vi "Python String to LabVIEW Data (Variant).vi"(6 "Data Type (for skipping type check)":T1 format="%.0x", 8 "error in (no error)":errorcluster, 9 "type":variant, 10 "Python String":string) -> (0 "error out":errorcluster, 2 "LabVIEW Data":variant)   [LabVIEW 2020, in "jki_python_data_tools.lvlib"]
uses:
  jki_python_data_tools.lvlib
  <userlib>/_OpenG.lib/string/string.llb/openg_string.lvlib
  <userlib>/_OpenG.lib/lvdata/lvdata.llb/openg_variant.lvlib
  <userlib>/_OpenG.lib/error/error.llb/openg_error.lvlib
  <userlib>/_OpenG.lib/lvdata/lvdata.llb/Type Descriptor Enumeration__ogtk.ctl
panel:
  # "Copyright © 2003-2009 JKI. All rights reserved.\n\nAuthor:\nPhilippe Guerit [philippe.guerit@jameskring.com]\nJim Kring [jim.kring@jameskring.com]\n\nThis library is provided \"AS IS\" ,WITHOUT WARRANTIES OR \nCONDITIONS OF ANY KIND, either express or implied.\n\nJames Kring, Inc. -- http://www.jameskring.com"
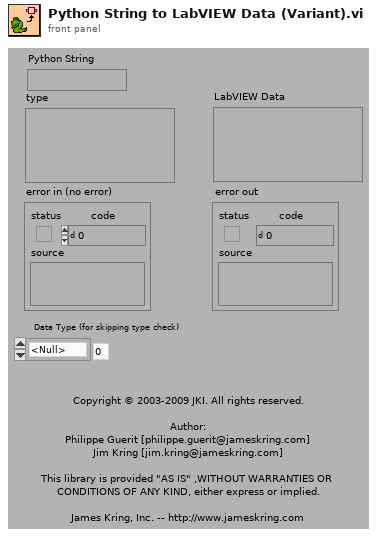
[diagram p1: front panel]
types:
  T1 = typedef "openg_variant.lvlib/Type Descriptor Enumeration__ogtk.ctl" = enum8{"<Null>", "I8", "I16", "I32", "I64", "U8", "U16", "U32", "U64", "SGL", "DBL", "EXT", "CSG", "CDB", "CXT", "0x0F", "0x10", "0x11", "0x12", "0x13", "0x14", "Enum U8", "Enum U16", "Enum U32", "Enum U64", "SGL PQ", "DBL PQ", "EXT PQ", "CSG PQ", "CDB PQ", "CXT PQ", "0x1F", "0x20", "Boolean", "0x22", "0x23", "0x24", "0x25", "0x26", "0x27", "0x28", "0x29", "0x2A", "0x2B", "0x2C", "0x2D", "0x2E", "0x2F", "String", "0x31", "Path", "Pict", "0x34", "0x35", "0x36", "DAQ", "0x38", "0x39", "0x3A", "0x3B", "0x3C", "0x3D", "0x3E", "0x3F", "Array", "0x41", "0x42", "0x43", "0x44", "0x45", "0x46", "0x47", "0x48", "0x49", "0x4A", "0x4B", "0x4C", "0x4D", "0x4E", "0x4F", "Cluster", "0x51", "0x52", "Variant", "Waveform", "0x55", "0x56", "0x57", "0x58", "0x59", "0x5A", "0x5B", "0x5C", "0x5D", "0x5E", "Fixed Point", "0x60", "0x61", "0x62", "0x63", "0x64", "0x65", "0x66", "0x67", "0x68", "0x69", "0x6A", "0x6B", "0x6C", "0x6D", "0x6E", "0x6F", "Refnum", "0x71", "0x72", "Set Collection", "Map Collection"}
  T2 = typedef "openg_variant.lvlib/Type Descriptor__ogtk.ctl" = i16[]
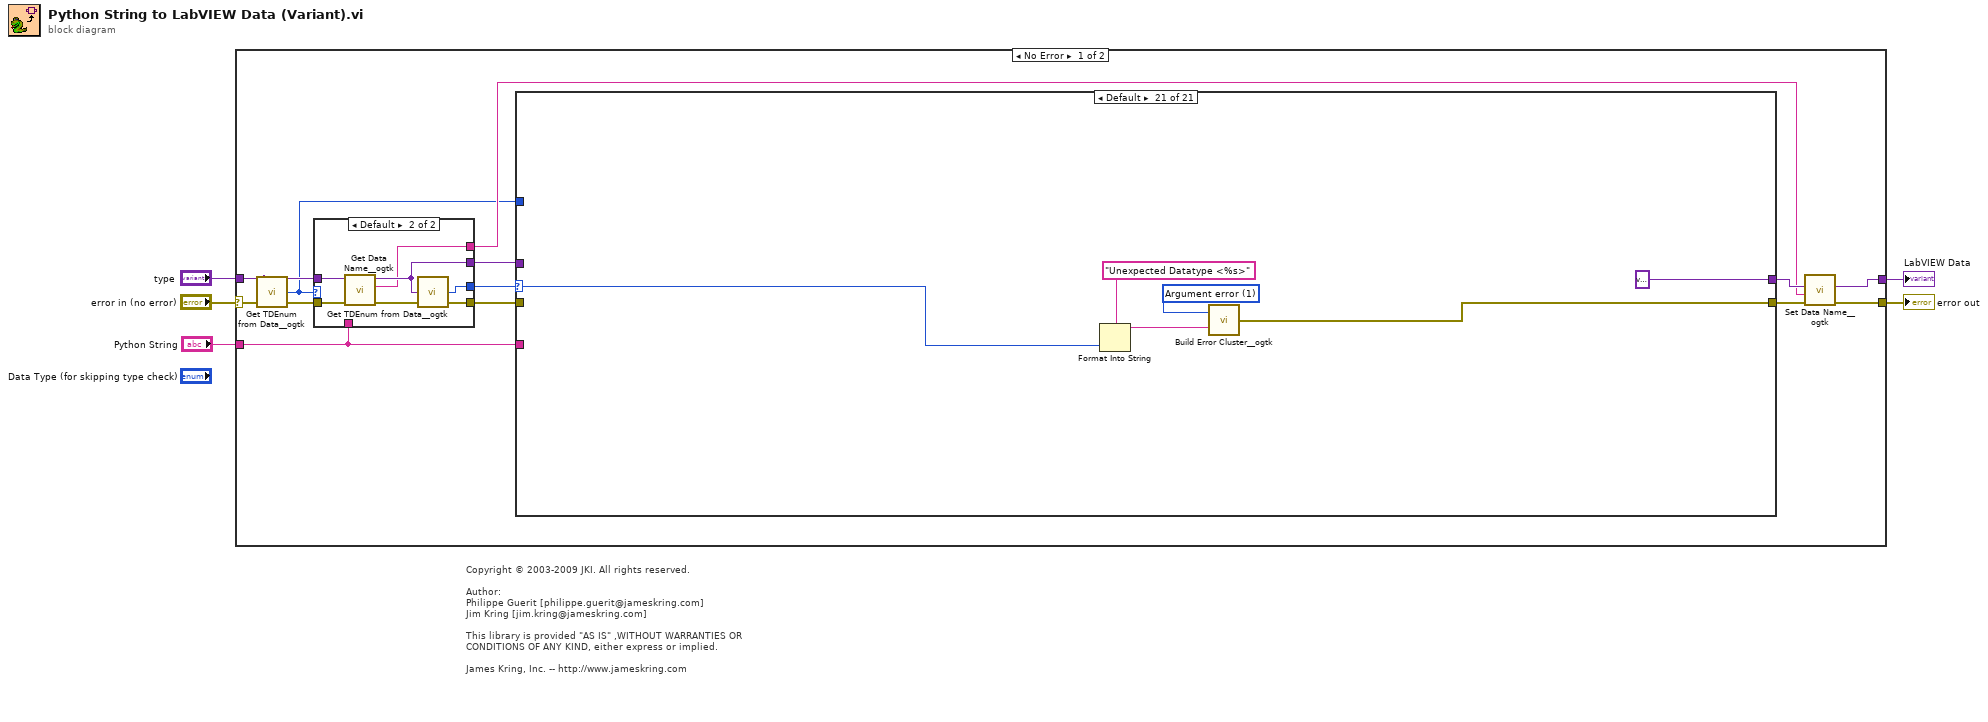
[diagram p0: block diagram]
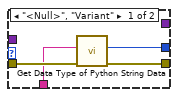
[diagram p2: hidden frame]
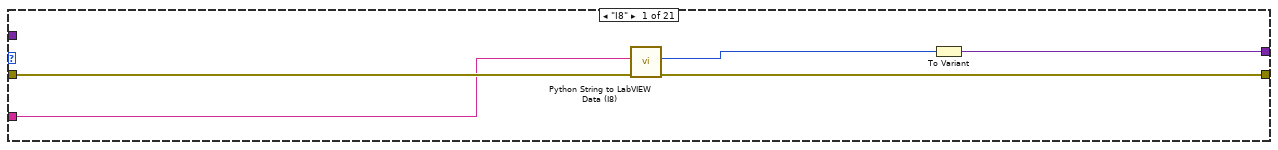
[diagram p3: hidden frame]
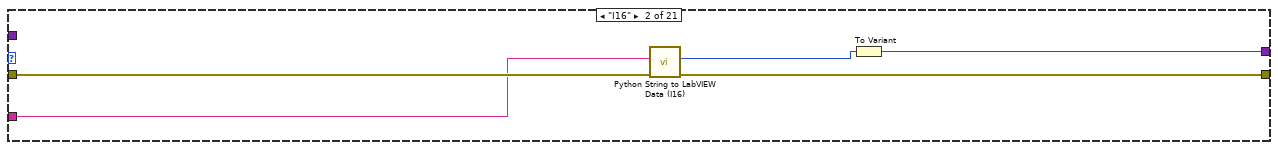
[diagram p4: hidden frame]
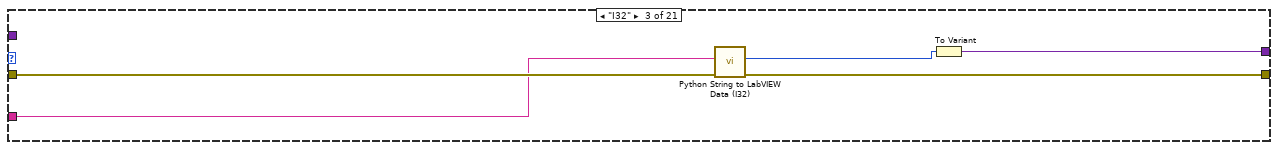
[diagram p5: hidden frame]
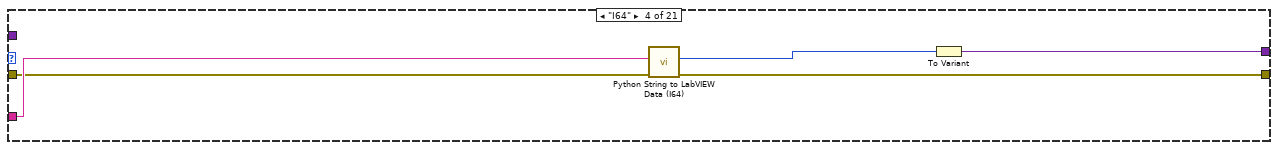
[diagram p6: hidden frame]
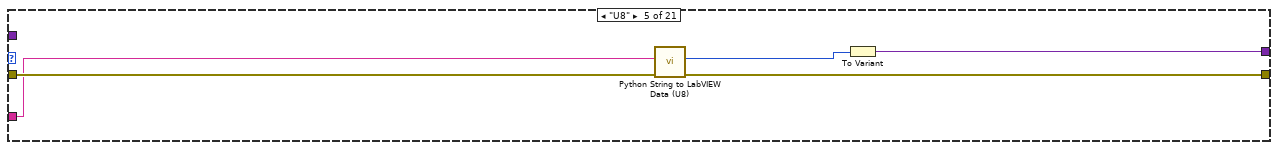
[diagram p7: hidden frame]
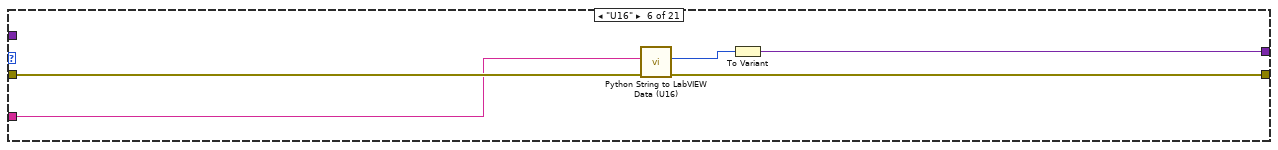
[diagram p8: hidden frame]
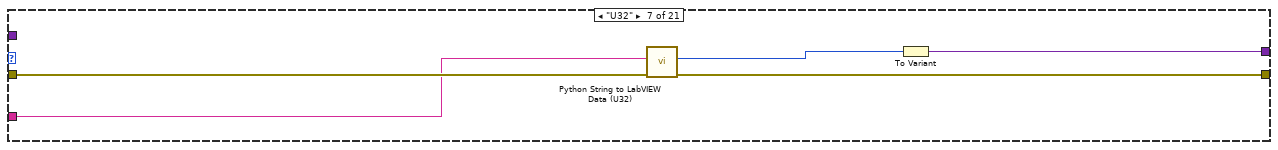
[diagram p9: hidden frame]
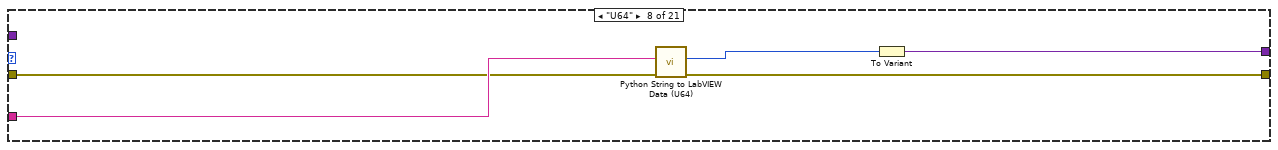
[diagram p10: hidden frame]
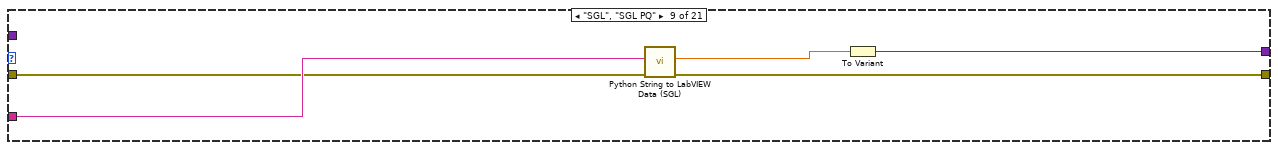
[diagram p11: hidden frame]
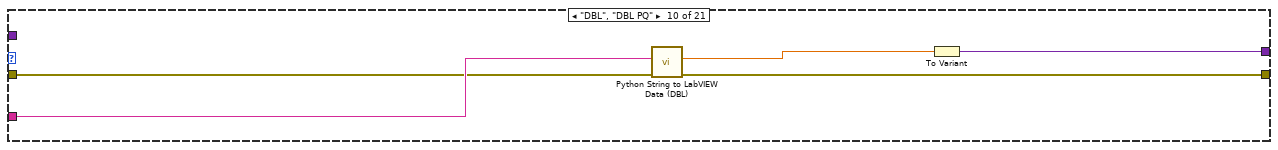
[diagram p12: hidden frame]
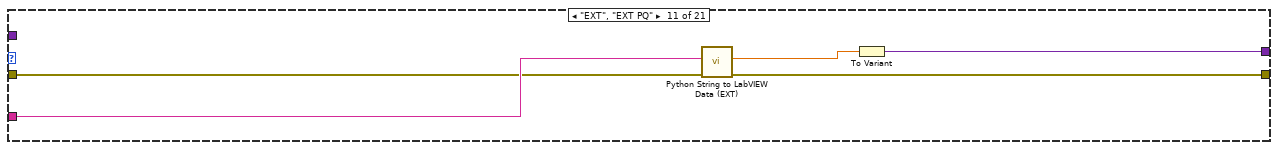
[diagram p13: hidden frame]
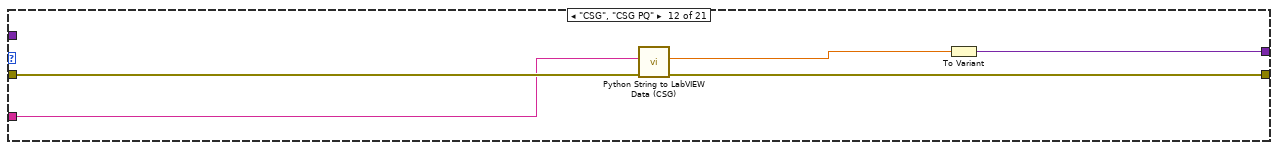
[diagram p14: hidden frame]
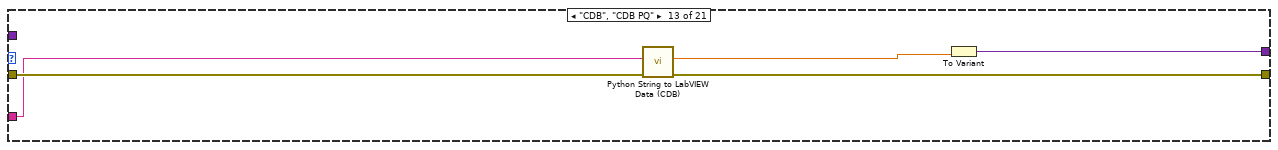
[diagram p15: hidden frame]
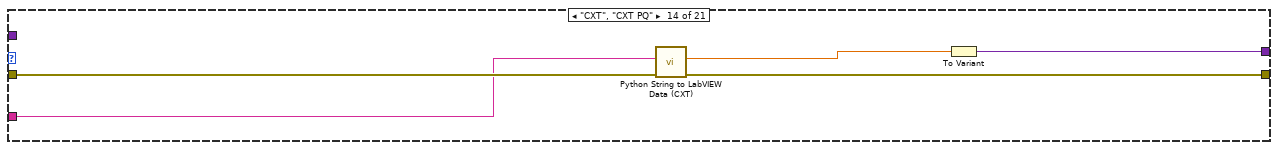
[diagram p16: hidden frame]
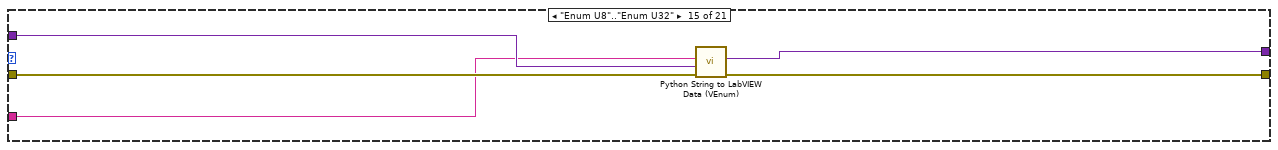
[diagram p17: hidden frame]
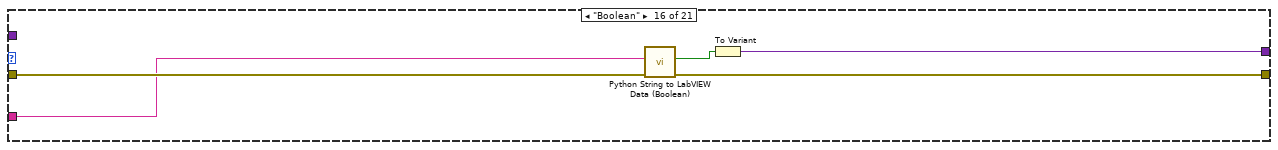
[diagram p18: hidden frame]
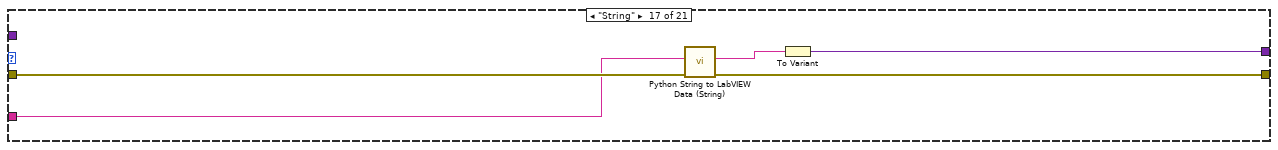
[diagram p19: hidden frame]
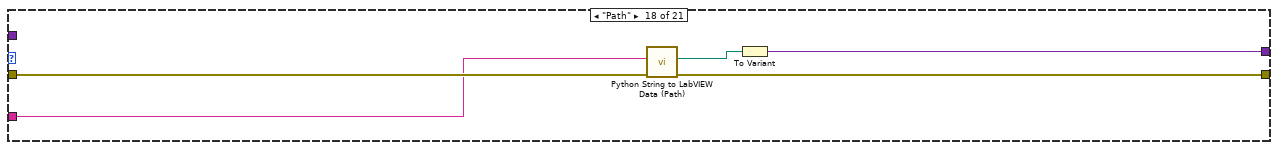
[diagram p20: hidden frame]
diagram:
  # "Copyright © 2003-2009 JKI. All rights reserved.\n\nAuthor:\nPhilippe Guerit [philippe.guerit@jameskring.com]\nJim Kring [jim.kring@jameskring.com]\n\nThis library is provided \"AS IS\" ,WITHOUT WARRANTIES OR \nCONDITIONS OF ANY KIND, either express or implied.\n\nJames Kring, Inc. -- http://www.jameskring.com"
  n1 = case shown="No Error" "error in (no error)" {
    selector: "error in (no error)" -> [w9 w756]
    tunnel: [w13 w756] -> w1
    tunnel: "type" -> [w8 _]
    tunnel: "Python String" -> [w7 _]
    tunnel: [w14 variant ("Variant")] -> w2
    frame No Error {
      n2 = call <userlib>:"Get TDEnum from Data__ogtk.vi"("Data"=w8) -> ("Type Descriptor Enumeration"=w6:T1)  [unwired: 4 in]
      n3 = case shown="Default" w6 {
        tunnel: [w18 w27] -> w17
        tunnel: [_ w26] -> w16
        tunnel: [w20 w25] -> w15
        tunnel: [_ w24] -> w10
        tunnel: w9 -> [w21 w23]
        tunnel: w8 -> [_ w22]
        tunnel: w7 -> [w19 _]
        frame "<Null>", "Variant" {
          n4 = call "Get Data Type of Python String Data.vi"("error in (no error)"=w21, "Python String"=w19) -> ("error out"=w20:errorcluster, "data type"=w18:T1)  [unwired: 8 in]
        }
        frame Default {
          n5 = call <userlib>:"Get Data Name__ogtk.vi"("error in (no error)"=w23, "Data"=w22) -> ("error out"=w25:errorcluster, "Data Name"=w24:string, "Data dup"=w26:variant)  [unwired: 7 in]
          n6 = call <userlib>:"Get TDEnum from Data__ogtk.vi"("Data"=w26) -> ("Type Descriptor Enumeration"=w27:T1)  [unwired: 4 in]
        }
      }
      n7 = case shown="Default" w17 {
        selector: w17 -> [_ _ _ _ _ _ _ _ _ _ _ _ _ _ _ _ _ _ _ _ w749]
        tunnel: w16 -> [_ _ _ _ _ _ _ _ _ _ _ _ _ _ w100 _ _ _ w121 w723 _]
        tunnel: [w30 w34 w40 w43 w48 w53 w60 w64 w70 w74 w79 w85 w89 w95 w101 w104 w108 w114 w119 w730 w753] -> w12
        tunnel: w15 -> [w32 w37 w41 w45 w51 w56 w61 w65 w68 w75 w80 w87 w92 w96 w102 w107 w112 w116 w120 w728 _]
        tunnel: [w31 w36 w42 w47 w52 w57 w62 w67 w72 w77 w82 w86 w91 w97 w99 w106 w111 w117 w118 w733 variant ("VCluster")] -> w11
        tunnel: w7 -> [w29 w33 w39 w46 w50 w55 w59 w66 w71 w76 w81 w83 w90 w94 w98 w105 w110 w113 w122 w729 _]
        tunnel: w6 -> [_ _ _ _ _ _ _ _ _ _ _ _ _ _ _ _ _ _ _ w725 _]
        frame "I8" {
          n8 = call "Python String to LabVIEW Data (I8).vi"("error in (no error)"=w32, "Python String"=w29) -> ("error out"=w30:errorcluster, "LabVIEW Data"=w28:i8)  [unwired: 8 in]
          n9 = To Variant(anything=w28) -> (Variant=w31:variant)
        }
        frame "I16" {
          n10 = call "Python String to LabVIEW Data (I16).vi"("error in (no error)"=w37, "Python String"=w33) -> ("error out"=w34:errorcluster, "LabVIEW Data"=w35:i16)  [unwired: 8 in]
          n11 = To Variant(anything=w35) -> (Variant=w36:variant)
        }
        frame "I32" {
          n12 = call "Python String to LabVIEW Data (I32).vi"("error in (no error)"=w41, "Python String"=w39) -> ("error out"=w40:errorcluster, "LabVIEW Data"=w38:i32)  [unwired: 8 in]
          n13 = To Variant(anything=w38) -> (Variant=w42:variant)
        }
        frame "I64" {
          n14 = call "Python String to LabVIEW Data (I64).vi"("error in (no error)"=w45, "Python String"=w46) -> ("error out"=w43:errorcluster, "LabVIEW Data"=w44:i64)  [unwired: 8 in]
          n15 = To Variant(anything=w44) -> (Variant=w47:variant)
        }
        frame "U8" {
          n16 = call "Python String to LabVIEW Data (U8).vi"("error in (no error)"=w51, "Python String"=w50) -> ("error out"=w48:errorcluster, "LabVIEW Data"=w49:u8)  [unwired: 8 in]
          n17 = To Variant(anything=w49) -> (Variant=w52:variant)
        }
        frame "U16" {
          n18 = call "Python String to LabVIEW Data (U16).vi"("error in (no error)"=w56, "Python String"=w55) -> ("error out"=w53:errorcluster, "LabVIEW Data"=w54:u16)  [unwired: 8 in]
          n19 = To Variant(anything=w54) -> (Variant=w57:variant)
        }
        frame "U32" {
          n20 = call "Python String to LabVIEW Data (U32).vi"("error in (no error)"=w61, "Python String"=w59) -> ("error out"=w60:errorcluster, "LabVIEW Data"=w58:u32)  [unwired: 8 in]
          n21 = To Variant(anything=w58) -> (Variant=w62:variant)
        }
        frame "U64" {
          n22 = call "Python String to LabVIEW Data (U64).vi"("error in (no error)"=w65, "Python String"=w66) -> ("error out"=w64:errorcluster, "LabVIEW Data"=w63:u64)  [unwired: 8 in]
          n23 = To Variant(anything=w63) -> (Variant=w67:variant)
        }
        frame "SGL", "SGL PQ" {
          n24 = call "Python String to LabVIEW Data (SGL).vi"("error in (no error)"=w68, "Python String"=w71) -> ("error out"=w70:errorcluster, "LabVIEW Data"=w69:sgl)  [unwired: 8 in]
          n25 = To Variant(anything=w69) -> (Variant=w72:variant)
        }
        frame "DBL", "DBL PQ" {
          n26 = call "Python String to LabVIEW Data (DBL).vi"("error in (no error)"=w75, "Python String"=w76) -> ("error out"=w74:errorcluster, "LabVIEW Data"=w73:dbl)  [unwired: 8 in]
          n27 = To Variant(anything=w73) -> (Variant=w77:variant)
        }
        frame "EXT", "EXT PQ" {
          n28 = call "Python String to LabVIEW Data (EXT).vi"("error in (no error)"=w80, "Python String"=w81) -> ("error out"=w79:errorcluster, "LabVIEW Data"=w78:ext)  [unwired: 8 in]
          n29 = To Variant(anything=w78) -> (Variant=w82:variant)
        }
        frame "CSG", "CSG PQ" {
          n30 = call "Python String to LabVIEW Data (CSG).vi"("error in (no error)"=w87, "Python String"=w83) -> ("error out"=w85:errorcluster, "LabVIEW Data"=w84:csg)  [unwired: 8 in]
          n31 = To Variant(anything=w84) -> (Variant=w86:variant)
        }
        frame "CDB", "CDB PQ" {
          n32 = call "Python String to LabVIEW Data (CDB).vi"("error in (no error)"=w92, "Python String"=w90) -> ("error out"=w89:errorcluster, "LabVIEW Data"=w88:cdb)  [unwired: 8 in]
          n33 = To Variant(anything=w88) -> (Variant=w91:variant)
        }
        frame "CXT", "CXT PQ" {
          n34 = call "Python String to LabVIEW Data (CXT).vi"("error in (no error)"=w96, "Python String"=w94) -> ("error out"=w95:errorcluster, "LabVIEW Data"=w93:cxt)  [unwired: 8 in]
          n35 = To Variant(anything=w93) -> (Variant=w97:variant)
        }
        frame "Enum U8".."Enum U32" {
          n36 = call "Python String to LabVIEW Data (VEnum).vi"("error in (no error)"=w102, "type (VEnum)"=w100, "Python String"=w98) -> ("error out"=w101:errorcluster, "LabVIEW Data"=w99:variant)  [unwired: 7 in]
        }
        frame "Boolean" {
          n37 = call "Python String to LabVIEW Data (Boolean).vi"("error in (no error)"=w107, "Python String"=w105) -> ("error out"=w104:errorcluster, "LabVIEW Data"=w103:bool)  [unwired: 8 in]
          n38 = To Variant(anything=w103) -> (Variant=w106:variant)
        }
        frame "String" {
          n39 = call "Python String to LabVIEW Data (String).vi"("error in (no error)"=w112, "Python String"=w110) -> ("error out"=w108:errorcluster, "LabVIEW Data"=w109:string)  [unwired: 8 in]
          n40 = To Variant(anything=w109) -> (Variant=w111:variant)
        }
        frame "Path" {
          n41 = call "Python String to LabVIEW Data (Path).vi"("error in (no error)"=w116, "Python String"=w113) -> ("error out"=w114:errorcluster, "LabVIEW Data"=w115:path)  [unwired: 8 in]
          n42 = To Variant(anything=w115) -> (Variant=w117:variant)
        }
        frame "Array" {
          n43 = disable-structure shown="Enabled" {
            disable-tunnel: w122 -> [w135 w166]
            disable-tunnel: w121 -> [w128 w170]
            disable-tunnel: w120 -> [w123 w174]
            disable-tunnel: [w125 w168] -> w119
            disable-tunnel: [w124 w167] -> w118
            frame Disabled {
              # "cluster or MutilD Array"
              # "Get Array Element\nvariant data type"
              # "/*Find opening \"[\" char*/"
              n44 = call <userlib>:"Get Array Element TDEnum__ogtk.vi"("error in (no error)"=w123, "Array"=w128) -> ("error out"=w134:errorcluster, "Element Type"=w126:T1)  [unwired: 8 in]
              n45 = call <userlib>:"Get Array Element TD__ogtk.vi"("error in (no error)"=w134, "Array"=w128) -> ("error out"=w133:errorcluster, "Type Descriptor"=w132:T2)  [unwired: 8 in]
              n46 = call "get text after first open bracket.vi"("Python String"=w135) -> ("Text After First Open Bracket"=w129:string)
              n47 = call <userlib>:"Get Default Data from TD__ogtk.vi"("error in (no error)"=w133, "Type Descriptor"=w132) -> ("error out"=w131:errorcluster, "Default VData"=w130:variant)  [unwired: 8 in]
              n48 = call "get text before last open bracket.vi"("Python String"=w129) -> ("Text After Last Open Bracket"=w127:string)
              n49 = case "Array Element Type" shown="\"Cluster\"" w126 {
                tunnel: w127 -> [w144 w160]
                tunnel: [w138 w157] -> w125
                tunnel: [w136 w156] -> w124
                tunnel: w130 -> [w137 w158]
                tunnel: w131 -> [w141 w159]
                frame "Cluster" {
                  n50 = call "Get Array Size from Python String.vi"("Python String"=w144) -> ("Array Size"=w142:i32, "Python String out"=w143:string)  [unwired: 9 in]
                  n51 = for "For each cluster element in the array" {
                    N: w142 -> [_]
                    tunnel: [w145] -> w140 mode=indexing
                    tunnel: w137 -> [w148]
                    shift-right: [w150] -> _
                    shift-left: w143 -> [w151]
                    shift-right: [w146] -> w139
                    shift-left: w141 -> [w147]
                    # "Recursive Call"
                    n52 = call "Split cluster or array pyhton string.vi"(11:w151) -> ("offset past element"=w150:i32, "First Element"=w149:string)  [unwired: 6 in, 3 out]
                    n53 = call "Python String to LabVIEW Data (Variant).vi"("error in (no error)"=w147, "type"=w148, "Python String"=w149) -> ("error out"=w146:errorcluster, "LabVIEW Data"=w145:variant)  [unwired: 7 in]
                  }
                  n54 = call <userlib>:"Array of VData to VArray__ogtk.vi"("error in (no error)"=w139, "Element Type (when empty)"=w137, "1D Array of VData"=w140) -> ("error out"=w138:errorcluster, "VArray"=w136:variant)  [unwired: 7 in]
                }
                frame Default {
                  # "Get Array Elements"
                  n55 = call <userlib>:"String to 1D Array__ogtk.vi"("delimiter (Tab)"=",", "string"=w160) -> ("Array of Strings"=w154:string[])  [unwired: 9 in]
                  n56 = for {
                    tunnel: w158 -> [w162]
                    tunnel: [w163] -> w153 mode=indexing
                    shift-right: [w164] -> w152
                    shift-left: w159 -> [w165]
                    tunnel: w154 -> [w161] mode=indexing
                    n57 = call "Python String to LabVIEW Data (Variant).vi"("error in (no error)"=w165, "type"=w162, "Python String"=w161) -> ("error out"=w164:errorcluster, "LabVIEW Data"=w163:variant)  [unwired: 7 in]
                  }
                  n58 = call <userlib>:"Array of VData to VArray__ogtk.vi"("error in (no error)"=w152, "Element Type (when empty)"=w158, "1D Array of VData"=w153) -> ("error out"=w157:errorcluster, "VArray"=w156:variant)  [unwired: 7 in]
                }
              }
            }
            frame Enabled {
              # "# of Dimensions"
              # "Get Array Element Type"
              n59 = call <userlib>:"Array Size(s)__ogtk.vi"("error in (no error)"=w174, "Array"=w170) -> ("error out"=w172:errorcluster, "N dims"=w173:u32)  [unwired: 7 in, 1 out]
              n60 = call <userlib>:"Get Array Element TDEnum__ogtk.vi"("error in (no error)"=w172, "Array"=w170) -> ("error out"=w171:errorcluster, "Element Type"=w169:T1)  [unwired: 8 in]
              n61 = case "Array dimension" shown="Default" w173 {
                tunnel: w170 -> [w181 w219 w368]
                tunnel: w171 -> [w176 w216 w363]
                tunnel: w169 -> [w182 w220 w369]
                tunnel: w166 -> [w178 w215 w365]
                tunnel: [w180 w218 w367] -> w168
                tunnel: [w179 w217 w366] -> w167
                frame Default {
                  # "Array of dim >= 2\nare not supported so put default code (that will failed) here for all array dim greater to 2"
                  n62 = call "Python List to Array of Elements.vi"("error in (no error)"=w176, "Python List"=w178) -> ("error out"=w175:errorcluster, "Elements"=w177:string[])  [unwired: 8 in]
                  n63 = case shown="Default" w182 {
                    tunnel: w175 -> [w187 w206]
                    tunnel: w181 -> [w185 w205]
                    tunnel: w177 -> [w183 w209]
                    tunnel: [w191 w199] -> w180
                    tunnel: [w190 w200] -> w179
                    frame Default {
                      # "Get Array Element\nvariant data type"
                      n64 = call <userlib>:"Get Array Element TD__ogtk.vi"("error in (no error)"=w187, "Array"=w185) -> ("error out"=w189:errorcluster, "Type Descriptor"=w188:T2)  [unwired: 8 in]
                      n65 = call <userlib>:"Get Default Data from TD__ogtk.vi"("error in (no error)"=w189, "Type Descriptor"=w188) -> ("error out"=w186:errorcluster, "Default VData"=w184:variant)  [unwired: 8 in]
                      n66 = for {
                        tunnel: w184 -> [w195]
                        tunnel: [w196] -> w193 mode=indexing
                        shift-right: [w197] -> w192
                        shift-left: w186 -> [w198]
                        tunnel: w183 -> [w194] mode=indexing
                        n67 = call "Python String to LabVIEW Data (Variant).vi"("error in (no error)"=w198, "type"=w195, "Python String"=w194) -> ("error out"=w197:errorcluster, "LabVIEW Data"=w196:variant)  [unwired: 7 in]
                      }
                      n68 = call <userlib>:"Array of VData to VArray__ogtk.vi"("error in (no error)"=w192, "Element Type (when empty)"=w184, "1D Array of VData"=w193) -> ("error out"=w191:errorcluster, "VArray"=w190:variant)  [unwired: 7 in]
                    }
                    frame "Cluster" {
                      # "Get Array Element\nvariant data type"
                      n69 = call <userlib>:"Get Array Element TD__ogtk.vi"("error in (no error)"=w206, "Array"=w205) -> ("error out"=w208:errorcluster, "Type Descriptor"=w207:T2)  [unwired: 8 in]
                      n70 = call <userlib>:"Get Default Data from TD__ogtk.vi"("error in (no error)"=w208, "Type Descriptor"=w207) -> ("error out"=w204:errorcluster, "Default VData"=w201:variant)  [unwired: 8 in]
                      n71 = for "For each cluster element in the array" {
                        tunnel: [w212] -> w202 mode=indexing
                        tunnel: w201 -> [w214]
                        shift-right: [w213] -> w203
                        shift-left: w204 -> [w210]
                        tunnel: w209 -> [w211] mode=indexing
                        # "Recursive Call"
                        n72 = call "Python String to LabVIEW Data (Variant).vi"("error in (no error)"=w210, "type"=w214, "Python String"=w211) -> ("error out"=w213:errorcluster, "LabVIEW Data"=w212:variant)  [unwired: 7 in]
                      }
                      n73 = call <userlib>:"Array of VData to VArray__ogtk.vi"("error in (no error)"=w203, "Element Type (when empty)"=w201, "1D Array of VData"=w202) -> ("error out"=w199:errorcluster, "VArray"=w200:variant)  [unwired: 7 in]
                    }
                  }
                }
                frame 1 {
                  # "1D array"
                  n74 = case shown="\"Cluster\"" w220 {
                    tunnel: w216 -> [w227 w243 w248 w251 w257 w262 w268 w272 w277 w282 w287 w292 w297 w302 w307 w313 w318 w323 w334]
                    tunnel: w219 -> [w226 _ _ _ _ _ _ _ _ _ _ _ _ _ _ _ _ _ w333]
                    tunnel: w215 -> [w224 w239 w244 w250 w256 w261 w264 w269 w274 w279 w284 w289 w294 w299 w304 w309 w314 w319 w327]
                    tunnel: [w231 w242 w247 w252 w258 w263 w267 w271 w276 w281 w286 w291 w296 w301 w306 w312 w317 w322 w328] -> w218
                    tunnel: [w230 w240 w245 w253 w254 w259 w265 w273 w278 w283 w288 w293 w298 w303 w308 w310 w315 w320 w329] -> w217
                    frame Default {
                      # "Get Array Element\nvariant data type"
                      n75 = call <userlib>:"Get Array Element TD__ogtk.vi"("error in (no error)"=w227, "Array"=w226) -> ("error out"=w229:errorcluster, "Type Descriptor"=w228:T2)  [unwired: 8 in]
                      n76 = call <userlib>:"Get Default Data from TD__ogtk.vi"("error in (no error)"=w229, "Type Descriptor"=w228) -> ("error out"=w222:errorcluster, "Default VData"=w225:variant)  [unwired: 8 in]
                      n77 = call "Python List to Array of Elements.vi"("error in (no error)"=w222, "Python List"=w224) -> ("error out"=w221:errorcluster, "Elements"=w223:string[])  [unwired: 8 in]
                      n78 = for {
                        tunnel: w225 -> [w235]
                        tunnel: [w236] -> w233 mode=indexing
                        shift-right: [w237] -> w232
                        shift-left: w221 -> [w238]
                        tunnel: w223 -> [w234] mode=indexing
                        n79 = call "Python String to LabVIEW Data (Variant).vi"("error in (no error)"=w238, "type"=w235, "Python String"=w234) -> ("error out"=w237:errorcluster, "LabVIEW Data"=w236:variant)  [unwired: 7 in]
                      }
                      n80 = call <userlib>:"Array of VData to VArray__ogtk.vi"("error in (no error)"=w232, "Element Type (when empty)"=w225, "1D Array of VData"=w233) -> ("error out"=w231:errorcluster, "VArray"=w230:variant)  [unwired: 7 in]
                    }
                    frame "I8" {
                      n81 = call "Python String to LabVIEW Data (I8 Array).vi"("error in (no error)"=w243, "Python String"=w239) -> ("error out"=w242:errorcluster, "LabVIEW Data"=w241:i8[])  [unwired: 8 in]
                      n82 = To Variant(anything=w241) -> (Variant=w240:variant)
                    }
                    frame "I16" {
                      n83 = call "Python String to LabVIEW Data (I16 Array).vi"("error in (no error)"=w248, "Python String"=w244) -> ("error out"=w247:errorcluster, "LabVIEW Data"=w246:i16[])  [unwired: 8 in]
                      n84 = To Variant(anything=w246) -> (Variant=w245:variant)
                    }
                    frame "I32" {
                      n85 = call "Python String to LabVIEW Data (I32 Array).vi"("error in (no error)"=w251, "Python String"=w250) -> ("error out"=w252:errorcluster, "LabVIEW Data"=w249:i32[])  [unwired: 8 in]
                      n86 = To Variant(anything=w249) -> (Variant=w253:variant)
                    }
                    frame "I64" {
                      n87 = call "Python String to LabVIEW Data (I64 Array).vi"("error in (no error)"=w257, "Python String"=w256) -> ("error out"=w258:errorcluster, "LabVIEW Data"=w255:i64[])  [unwired: 8 in]
                      n88 = To Variant(anything=w255) -> (Variant=w254:variant)
                    }
                    frame "U8" {
                      n89 = call "Python String to LabVIEW Data (U8 Array).vi"("error in (no error)"=w262, "Python String"=w261) -> ("error out"=w263:errorcluster, "LabVIEW Data"=w260:u8[])  [unwired: 8 in]
                      n90 = To Variant(anything=w260) -> (Variant=w259:variant)
                    }
                    frame "U16" {
                      n91 = call "Python String to LabVIEW Data (U16 Array).vi"("error in (no error)"=w268, "Python String"=w264) -> ("error out"=w267:errorcluster, "LabVIEW Data"=w266:u16[])  [unwired: 8 in]
                      n92 = To Variant(anything=w266) -> (Variant=w265:variant)
                    }
                    frame "U32" {
                      n93 = call "Python String to LabVIEW Data (U32 Array).vi"("error in (no error)"=w272, "Python String"=w269) -> ("error out"=w271:errorcluster, "LabVIEW Data"=w270:u32[])  [unwired: 8 in]
                      n94 = To Variant(anything=w270) -> (Variant=w273:variant)
                    }
                    frame "U64" {
                      n95 = call "Python String to LabVIEW Data (U64 Array).vi"("error in (no error)"=w277, "Python String"=w274) -> ("error out"=w276:errorcluster, "LabVIEW Data"=w275:u64[])  [unwired: 8 in]
                      n96 = To Variant(anything=w275) -> (Variant=w278:variant)
                    }
                    frame "SGL", "SGL PQ" {
                      n97 = call "Python String to LabVIEW Data (SGL Array).vi"("error in (no error)"=w282, "Python String"=w279) -> ("error out"=w281:errorcluster, "LabVIEW Data"=w280:sgl[])  [unwired: 8 in]
                      n98 = To Variant(anything=w280) -> (Variant=w283:variant)
                    }
                    frame "DBL", "DBL PQ" {
                      n99 = call "Python String to LabVIEW Data (DBL Array).vi"("error in (no error)"=w287, "Python String"=w284) -> ("error out"=w286:errorcluster, "LabVIEW Data"=w285:dbl[])  [unwired: 8 in]
                      n100 = To Variant(anything=w285) -> (Variant=w288:variant)
                    }
                    frame "EXT", "EXT PQ" {
                      n101 = call "Python String to LabVIEW Data (EXT Array).vi"("error in (no error)"=w292, "Python String"=w289) -> ("error out"=w291:errorcluster, "LabVIEW Data"=w290:ext[])  [unwired: 8 in]
                      n102 = To Variant(anything=w290) -> (Variant=w293:variant)
                    }
                    frame "CSG", "CSG PQ" {
                      n103 = call "Python String to LabVIEW Data (CSG Array).vi"("error in (no error)"=w297, "Python String"=w294) -> ("error out"=w296:errorcluster, "LabVIEW Data"=w295:csg[])  [unwired: 8 in]
                      n104 = To Variant(anything=w295) -> (Variant=w298:variant)
                    }
                    frame "CDB", "CDB PQ" {
                      n105 = call "Python String to LabVIEW Data (CDB Array).vi"("error in (no error)"=w302, "Python String"=w299) -> ("error out"=w301:errorcluster, "LabVIEW Data"=w300:cdb[])  [unwired: 8 in]
                      n106 = To Variant(anything=w300) -> (Variant=w303:variant)
                    }
                    frame "CXT", "CXT PQ" {
                      n107 = call "Python String to LabVIEW Data (CXT Array).vi"("error in (no error)"=w307, "Python String"=w304) -> ("error out"=w306:errorcluster, "LabVIEW Data"=w305:cxt[])  [unwired: 8 in]
                      n108 = To Variant(anything=w305) -> (Variant=w308:variant)
                    }
                    frame "Boolean" {
                      n109 = call "Python String to LabVIEW Data (Boolean Array).vi"("error in (no error)"=w313, "Python String"=w309) -> ("error out"=w312:errorcluster, "LabVIEW Data"=w311:bool[])  [unwired: 8 in]
                      n110 = To Variant(anything=w311) -> (Variant=w310:variant)
                    }
                    frame "String" {
                      n111 = call "Python String to LabVIEW Data (String Array).vi"("error in (no error)"=w318, "Python String"=w314) -> ("error out"=w317:errorcluster, "LabVIEW Data"=w316:string[])  [unwired: 8 in]
                      n112 = To Variant(anything=w316) -> (Variant=w315:variant)
                    }
                    frame "Path" {
                      n113 = call "Python String to LabVIEW Data (Path Array).vi"("error in (no error)"=w323, "Python String"=w319) -> ("error out"=w322:errorcluster, "LabVIEW Data"=w321:path[])  [unwired: 8 in]
                      n114 = To Variant(anything=w321) -> (Variant=w320:variant)
                    }
                    frame "Cluster" {
                      # "Get Array Element\nvariant data type"
                      n115 = call <userlib>:"Get Array Element TD__ogtk.vi"("error in (no error)"=w334, "Array"=w333) -> ("error out"=w336:errorcluster, "Type Descriptor"=w335:T2)  [unwired: 8 in]
                      n116 = call <userlib>:"Get Default Data from TD__ogtk.vi"("error in (no error)"=w336, "Type Descriptor"=w335) -> ("error out"=w325:errorcluster, "Default VData"=w330:variant)  [unwired: 8 in]
                      n117 = call "Python List to Array of Elements.vi"("error in (no error)"=w325, "Python List"=w327) -> ("error out"=w324:errorcluster, "Elements"=w326:string[])  [unwired: 8 in]
                      n118 = disable-structure shown="Disabled" {
                        disable-tunnel: w326 -> [w342 w352 _]
                        disable-tunnel: w324 -> [w341 w356 _]
                        disable-tunnel: [w340 w355 _] -> w332
                        disable-tunnel: [w339 w354 _] -> w331
                        disable-tunnel: w330 -> [w338 w353 _]
                        frame Disabled {
                          n119 = call "get text between brackets.vi"("Python String"=w342) -> ("Text Between Brakets"=w337:string)  [unwired: 10 in]
                          n120 = call "Get Array Size from Python String.vi"("Python String"=w337) -> ("Array Size"=w343:i32, "Python String out"=w344:string)  [unwired: 9 in]
                          n121 = for "For each cluster element in the array" {
                            N: w343 -> [_]
                            tunnel: [w345] -> w339 mode=indexing
                            tunnel: w338 -> [w348]
                            shift-right: [w350] -> _
                            shift-left: w344 -> [w351]
                            shift-right: [w346] -> w340
                            shift-left: w341 -> [w347]
                            # "Recursive Call"
                            n122 = call "Split cluster or array pyhton string.vi"(11:w351) -> ("offset past element"=w350:i32, "First Element"=w349:string)  [unwired: 6 in, 3 out]
                            n123 = call "Python String to LabVIEW Data (Variant).vi"("error in (no error)"=w347, "type"=w348, "Python String"=w349) -> ("error out"=w346:errorcluster, "LabVIEW Data"=w345:variant)  [unwired: 7 in]
                          }
                        }
                        frame Enabled {
                          n124 = for "For each cluster element in the array" {
                            tunnel: [w359] -> w354 mode=indexing
                            tunnel: w353 -> [w361]
                            shift-right: [w360] -> w355
                            shift-left: w356 -> [w357]
                            tunnel: w352 -> [w358] mode=indexing
                            # "Recursive Call"
                            n125 = call "Python String to LabVIEW Data (Variant).vi"("error in (no error)"=w357, "type"=w361, "Python String"=w358) -> ("error out"=w360:errorcluster, "LabVIEW Data"=w359:variant)  [unwired: 7 in]
                          }
                        }
                        frame Disabled {
                        }
                      }
                      n126 = call <userlib>:"Array of VData to VArray__ogtk.vi"("error in (no error)"=w332, "Element Type (when empty)"=w330, "1D Array of VData"=w331) -> ("error out"=w328:errorcluster, "VArray"=w329:variant)  [unwired: 7 in]
                    }
                  }
                }
                frame 2 {
                  # "2D array"
                  n127 = call "Python List to Array of Elements.vi"("error in (no error)"=w363, "Python List"=w365) -> ("error out"=w362:errorcluster, "Elements"=w364:string[])  [unwired: 8 in]
                  n128 = case shown="\"I8\"" w369 {
                    tunnel: w362 -> [w380 w395 w409 w429 w446 w463 w480 w497 w514 w531 w548 w565 w582 w599 w616 w633 w650 w667 w688]
                    tunnel: w368 -> [w379 _ _ _ _ _ _ _ _ _ _ _ _ _ _ _ _ _ w687]
                    tunnel: [w377 w394 w412 w428 w445 w462 w479 w496 w513 w530 w547 w564 w581 w598 w615 w632 w649 w666 w684] -> w367
                    tunnel: [w376 w392 w410 w426 w443 w460 w477 w494 w511 w528 w545 w562 w579 w596 w613 w630 w647 w664 w682] -> w366
                    tunnel: w364 -> [w370 w391 w408 w425 w442 w459 w476 w493 w510 w527 w544 w561 w578 w595 w612 w629 w646 w663 w681]
                    frame Default {
                      # "Get Array Element\nvariant data type"
                      n129 = call <userlib>:"Get Array Element TD__ogtk.vi"("error in (no error)"=w380, "Array"=w379) -> ("error out"=w382:errorcluster, "Type Descriptor"=w381:T2)  [unwired: 8 in]
                      n130 = call <userlib>:"Get Default Data from TD__ogtk.vi"("error in (no error)"=w382, "Type Descriptor"=w381) -> ("error out"=w371:errorcluster, "Default VData"=w374:variant)  [unwired: 8 in]
                      n131 = Build Array(w374) -> (w375:variant[])
                      n132 = call <userlib>:"Array of VData to VArray__ogtk.vi"("error in (no error)"=w371, "Element Type (when empty)"=w374, "1D Array of VData"=w375) -> ("error out"=w372:errorcluster, "VArray"=w373:variant)  [unwired: 7 in]
                      n133 = for {
                        tunnel: w373 -> [w389]
                        shift-right: [w386] -> w377
                        shift-left: w372 -> [w390]
                        tunnel: [w384] -> w378 mode=indexing
                        tunnel: w370 -> [w383] mode=indexing
                        n134 = call "Python String to LabVIEW Data (Variant).vi"("error in (no error)"=w390, "type"=w389, "Python String"=w383) -> ("error out"=w387:errorcluster, "LabVIEW Data"=w388:variant)  [unwired: 7 in]
                        n135 = Variant To Data(error in=w387, type=variant[] [], Variant=w388) -> (data=w384:variant[], error out=w386:errorcluster)
                      }
                      n136 = To Variant(anything=w378) -> (Variant=w376:variant)
                    }
                    frame "I8" {
                      n137 = for {
                        tunnel: [w401] -> w393 mode=indexing
                        shift-right: [w402] -> w394
                        shift-left: w395 -> [w398]
                        tunnel: w391 -> [w397] mode=indexing
                        # "Get Array Elements"
                        n138 = call "get text between brackets.vi"("Python String"=w397) -> ("Text Between Brakets"=w396:string)  [unwired: 10 in]
                        n139 = call <userlib>:"String to 1D Array__ogtk.vi"("delimiter (Tab)"=",", "string"=w396) -> ("Array of Strings"=w399:string[])  [unwired: 9 in]
                        n140 = for {
                          tunnel: [w403] -> w401 mode=indexing
                          tunnel: w399 -> [w404] mode=indexing
                          shift-right: [w406] -> w402
                          shift-left: w398 -> [w407]
                          w405 = i8 0  # I8 Type
                          n141 = Scan From String(input string=w404, error in=w407, default 1=w405) -> (error out=w406:errorcluster, output 1=w403:i8)  [unwired: 2 in, 2 out]
                        }
                      }
                      n142 = To Variant(anything=w393) -> (Variant=w392:variant)
                    }
                    frame "I16" {
                      n143 = for {
                        tunnel: [w417] -> w411 mode=indexing
                        tunnel: w408 -> [w414] mode=indexing
                        shift-right: [w418] -> w412
                        shift-left: w409 -> [w419]
                        # "Get Array Elements"
                        n144 = call "get text between brackets.vi"("Python String"=w414) -> ("Text Between Brakets"=w413:string)  [unwired: 10 in]
                        n145 = call <userlib>:"String to 1D Array__ogtk.vi"("delimiter (Tab)"=",", "string"=w413) -> ("Array of Strings"=w415:string[])  [unwired: 9 in]
                        n146 = for {
                          tunnel: [w420] -> w417 mode=indexing
                          tunnel: w415 -> [w421] mode=indexing
                          shift-right: [w423] -> w418
                          shift-left: w419 -> [w424]
                          w422 = i16 0  # I16 Type
                          n147 = Scan From String(input string=w421, error in=w424, default 1=w422) -> (error out=w423:errorcluster, output 1=w420:i16)  [unwired: 2 in, 2 out]
                        }
                      }
                      n148 = To Variant(anything=w411) -> (Variant=w410:variant)
                    }
                    frame "I32" {
                      n149 = for {
                        tunnel: [w434] -> w427 mode=indexing
                        tunnel: w425 -> [w431] mode=indexing
                        shift-right: [w435] -> w428
                        shift-left: w429 -> [w436]
                        # "Get Array Elements"
                        n150 = call "get text between brackets.vi"("Python String"=w431) -> ("Text Between Brakets"=w430:string)  [unwired: 10 in]
                        n151 = call <userlib>:"String to 1D Array__ogtk.vi"("delimiter (Tab)"=",", "string"=w430) -> ("Array of Strings"=w432:string[])  [unwired: 9 in]
                        n152 = for {
                          tunnel: [w437] -> w434 mode=indexing
                          tunnel: w432 -> [w438] mode=indexing
                          shift-right: [w440] -> w435
                          shift-left: w436 -> [w441]
                          w439 = 0  # I32 Type
                          n153 = Scan From String(input string=w438, error in=w441, default 1=w439) -> (error out=w440:errorcluster, output 1=w437:i32)  [unwired: 2 in, 2 out]
                        }
                      }
                      n154 = To Variant(anything=w427) -> (Variant=w426:variant)
                    }
                    frame "I64" {
                      n155 = for {
                        tunnel: [w451] -> w444 mode=indexing
                        tunnel: w442 -> [w448] mode=indexing
                        shift-right: [w452] -> w445
                        shift-left: w446 -> [w453]
                        # "Get Array Elements"
                        n156 = call "get text between brackets.vi"("Python String"=w448) -> ("Text Between Brakets"=w447:string)  [unwired: 10 in]
                        n157 = call <userlib>:"String to 1D Array__ogtk.vi"("delimiter (Tab)"=",", "string"=w447) -> ("Array of Strings"=w449:string[])  [unwired: 9 in]
                        n158 = for {
                          tunnel: [w454] -> w451 mode=indexing
                          tunnel: w449 -> [w455] mode=indexing
                          shift-right: [w457] -> w452
                          shift-left: w453 -> [w458]
                          w456 = i64 0  # I64 Type
                          n159 = Scan From String(input string=w455, error in=w458, default 1=w456) -> (error out=w457:errorcluster, output 1=w454:i64)  [unwired: 2 in, 2 out]
                        }
                      }
                      n160 = To Variant(anything=w444) -> (Variant=w443:variant)
                    }
                    frame "U8" {
                      n161 = for {
                        tunnel: [w468] -> w461 mode=indexing
                        tunnel: w459 -> [w465] mode=indexing
                        shift-right: [w469] -> w462
                        shift-left: w463 -> [w470]
                        # "Get Array Elements"
                        n162 = call "get text between brackets.vi"("Python String"=w465) -> ("Text Between Brakets"=w464:string)  [unwired: 10 in]
                        n163 = call <userlib>:"String to 1D Array__ogtk.vi"("delimiter (Tab)"=",", "string"=w464) -> ("Array of Strings"=w466:string[])  [unwired: 9 in]
                        n164 = for {
                          tunnel: [w471] -> w468 mode=indexing
                          tunnel: w466 -> [w472] mode=indexing
                          shift-right: [w474] -> w469
                          shift-left: w470 -> [w475]
                          w473 = u8 0  # U8 Type
                          n165 = Scan From String(input string=w472, error in=w475, default 1=w473) -> (error out=w474:errorcluster, output 1=w471:u8)  [unwired: 2 in, 2 out]
                        }
                      }
                      n166 = To Variant(anything=w461) -> (Variant=w460:variant)
                    }
                    frame "U16" {
                      n167 = for {
                        tunnel: [w485] -> w478 mode=indexing
                        tunnel: w476 -> [w482] mode=indexing
                        shift-right: [w486] -> w479
                        shift-left: w480 -> [w487]
                        # "Get Array Elements"
                        n168 = call "get text between brackets.vi"("Python String"=w482) -> ("Text Between Brakets"=w481:string)  [unwired: 10 in]
                        n169 = call <userlib>:"String to 1D Array__ogtk.vi"("delimiter (Tab)"=",", "string"=w481) -> ("Array of Strings"=w483:string[])  [unwired: 9 in]
                        n170 = for {
                          tunnel: [w488] -> w485 mode=indexing
                          tunnel: w483 -> [w489] mode=indexing
                          shift-right: [w491] -> w486
                          shift-left: w487 -> [w492]
                          w490 = u16 0  # U16 Type
                          n171 = Scan From String(input string=w489, error in=w492, default 1=w490) -> (error out=w491:errorcluster, output 1=w488:u16)  [unwired: 2 in, 2 out]
                        }
                      }
                      n172 = To Variant(anything=w478) -> (Variant=w477:variant)
                    }
                    frame "U32" {
                      n173 = for {
                        tunnel: [w502] -> w495 mode=indexing
                        tunnel: w493 -> [w499] mode=indexing
                        shift-right: [w503] -> w496
                        shift-left: w497 -> [w504]
                        # "Get Array Elements"
                        n174 = call "get text between brackets.vi"("Python String"=w499) -> ("Text Between Brakets"=w498:string)  [unwired: 10 in]
                        n175 = call <userlib>:"String to 1D Array__ogtk.vi"("delimiter (Tab)"=",", "string"=w498) -> ("Array of Strings"=w500:string[])  [unwired: 9 in]
                        n176 = for {
                          tunnel: [w505] -> w502 mode=indexing
                          tunnel: w500 -> [w506] mode=indexing
                          shift-right: [w508] -> w503
                          shift-left: w504 -> [w509]
                          w507 = u32 0  # U32 Type
                          n177 = Scan From String(input string=w506, error in=w509, default 1=w507) -> (error out=w508:errorcluster, output 1=w505:u32)  [unwired: 2 in, 2 out]
                        }
                      }
                      n178 = To Variant(anything=w495) -> (Variant=w494:variant)
                    }
                    frame "U64" {
                      n179 = for {
                        tunnel: [w519] -> w512 mode=indexing
                        tunnel: w510 -> [w516] mode=indexing
                        shift-right: [w520] -> w513
                        shift-left: w514 -> [w521]
                        # "Get Array Elements"
                        n180 = call "get text between brackets.vi"("Python String"=w516) -> ("Text Between Brakets"=w515:string)  [unwired: 10 in]
                        n181 = call <userlib>:"String to 1D Array__ogtk.vi"("delimiter (Tab)"=",", "string"=w515) -> ("Array of Strings"=w517:string[])  [unwired: 9 in]
                        n182 = for {
                          tunnel: [w522] -> w519 mode=indexing
                          tunnel: w517 -> [w523] mode=indexing
                          shift-right: [w525] -> w520
                          shift-left: w521 -> [w526]
                          w524 = u64 0  # U64 Type
                          n183 = Scan From String(input string=w523, error in=w526, default 1=w524) -> (error out=w525:errorcluster, output 1=w522:u64)  [unwired: 2 in, 2 out]
                        }
                      }
                      n184 = To Variant(anything=w512) -> (Variant=w511:variant)
                    }
                    frame "SGL", "SGL PQ" {
                      n185 = for {
                        tunnel: [w536] -> w529 mode=indexing
                        tunnel: w527 -> [w533] mode=indexing
                        shift-right: [w537] -> w530
                        shift-left: w531 -> [w538]
                        # "Get Array Elements"
                        n186 = call "get text between brackets.vi"("Python String"=w533) -> ("Text Between Brakets"=w532:string)  [unwired: 10 in]
                        n187 = call <userlib>:"String to 1D Array__ogtk.vi"("delimiter (Tab)"=",", "string"=w532) -> ("Array of Strings"=w534:string[])  [unwired: 9 in]
                        n188 = for {
                          tunnel: [w539] -> w536 mode=indexing
                          tunnel: w534 -> [w540] mode=indexing
                          shift-right: [w542] -> w537
                          shift-left: w538 -> [w543]
                          w541 = sgl 0.0  # SGL Type
                          n189 = Scan From String(input string=w540, error in=w543, default 1=w541) -> (error out=w542:errorcluster, output 1=w539:sgl)  [unwired: 2 in, 2 out]
                        }
                      }
                      n190 = To Variant(anything=w529) -> (Variant=w528:variant)
                    }
                    frame "DBL", "DBL PQ" {
                      n191 = for {
                        tunnel: [w553] -> w546 mode=indexing
                        tunnel: w544 -> [w550] mode=indexing
                        shift-right: [w554] -> w547
                        shift-left: w548 -> [w555]
                        # "Get Array Elements"
                        n192 = call "get text between brackets.vi"("Python String"=w550) -> ("Text Between Brakets"=w549:string)  [unwired: 10 in]
                        n193 = call <userlib>:"String to 1D Array__ogtk.vi"("delimiter (Tab)"=",", "string"=w549) -> ("Array of Strings"=w551:string[])  [unwired: 9 in]
                        n194 = for {
                          tunnel: [w556] -> w553 mode=indexing
                          tunnel: w551 -> [w557] mode=indexing
                          shift-right: [w559] -> w554
                          shift-left: w555 -> [w560]
                          w558 = 0.0  # DBL Type
                          n195 = Scan From String(input string=w557, error in=w560, default 1=w558) -> (error out=w559:errorcluster, output 1=w556:dbl)  [unwired: 2 in, 2 out]
                        }
                      }
                      n196 = To Variant(anything=w546) -> (Variant=w545:variant)
                    }
                    frame "EXT", "EXT PQ" {
                      n197 = for {
                        tunnel: [w570] -> w563 mode=indexing
                        tunnel: w561 -> [w567] mode=indexing
                        shift-right: [w571] -> w564
                        shift-left: w565 -> [w572]
                        # "Get Array Elements"
                        n198 = call "get text between brackets.vi"("Python String"=w567) -> ("Text Between Brakets"=w566:string)  [unwired: 10 in]
                        n199 = call <userlib>:"String to 1D Array__ogtk.vi"("delimiter (Tab)"=",", "string"=w566) -> ("Array of Strings"=w568:string[])  [unwired: 9 in]
                        n200 = for {
                          tunnel: [w573] -> w570 mode=indexing
                          tunnel: w568 -> [w574] mode=indexing
                          shift-right: [w576] -> w571
                          shift-left: w572 -> [w577]
                          w575 = ext 0.0  # EXT Type
                          n201 = Scan From String(input string=w574, error in=w577, default 1=w575) -> (error out=w576:errorcluster, output 1=w573:ext)  [unwired: 2 in, 2 out]
                        }
                      }
                      n202 = To Variant(anything=w563) -> (Variant=w562:variant)
                    }
                    frame "CSG", "CSG PQ" {
                      n203 = for {
                        tunnel: [w587] -> w580 mode=indexing
                        tunnel: w578 -> [w584] mode=indexing
                        shift-right: [w588] -> w581
                        shift-left: w582 -> [w589]
                        # "Get Array Elements"
                        n204 = call "get text between brackets.vi"("Python String"=w584) -> ("Text Between Brakets"=w583:string)  [unwired: 10 in]
                        n205 = call <userlib>:"String to 1D Array__ogtk.vi"("delimiter (Tab)"=",", "string"=w583) -> ("Array of Strings"=w585:string[])  [unwired: 9 in]
                        n206 = for {
                          tunnel: [w590] -> w587 mode=indexing
                          tunnel: w585 -> [w591] mode=indexing
                          shift-right: [w593] -> w588
                          shift-left: w589 -> [w594]
                          w592 = csg 0.0+0.0i  # CSG Type
                          n207 = Scan From String(input string=w591, error in=w594, default 1=w592) -> (error out=w593:errorcluster, output 1=w590:csg)  [unwired: 2 in, 2 out]
                        }
                      }
                      n208 = To Variant(anything=w580) -> (Variant=w579:variant)
                    }
                    frame "CDB", "CDB PQ" {
                      n209 = for {
                        tunnel: [w604] -> w597 mode=indexing
                        tunnel: w595 -> [w601] mode=indexing
                        shift-right: [w605] -> w598
                        shift-left: w599 -> [w606]
                        # "Get Array Elements"
                        n210 = call "get text between brackets.vi"("Python String"=w601) -> ("Text Between Brakets"=w600:string)  [unwired: 10 in]
                        n211 = call <userlib>:"String to 1D Array__ogtk.vi"("delimiter (Tab)"=",", "string"=w600) -> ("Array of Strings"=w602:string[])  [unwired: 9 in]
                        n212 = for {
                          tunnel: [w607] -> w604 mode=indexing
                          tunnel: w602 -> [w608] mode=indexing
                          shift-right: [w610] -> w605
                          shift-left: w606 -> [w611]
                          w609 = cdb 0.0+0.0i  # CDB Type
                          n213 = Scan From String(input string=w608, error in=w611, default 1=w609) -> (error out=w610:errorcluster, output 1=w607:cdb)  [unwired: 2 in, 2 out]
                        }
                      }
                      n214 = To Variant(anything=w597) -> (Variant=w596:variant)
                    }
                    frame "CXT", "CXT PQ" {
                      n215 = for {
                        tunnel: [w621] -> w614 mode=indexing
                        tunnel: w612 -> [w618] mode=indexing
                        shift-right: [w622] -> w615
                        shift-left: w616 -> [w623]
                        # "Get Array Elements"
                        n216 = call "get text between brackets.vi"("Python String"=w618) -> ("Text Between Brakets"=w617:string)  [unwired: 10 in]
                        n217 = call <userlib>:"String to 1D Array__ogtk.vi"("delimiter (Tab)"=",", "string"=w617) -> ("Array of Strings"=w619:string[])  [unwired: 9 in]
                        n218 = for {
                          tunnel: [w624] -> w621 mode=indexing
                          tunnel: w619 -> [w625] mode=indexing
                          shift-right: [w627] -> w622
                          shift-left: w623 -> [w628]
                          w626 = cxt 0.0+0.0i  # CXT Type
                          n219 = Scan From String(input string=w625, error in=w628, default 1=w626) -> (error out=w627:errorcluster, output 1=w624:cxt)  [unwired: 2 in, 2 out]
                        }
                      }
                      n220 = To Variant(anything=w614) -> (Variant=w613:variant)
                    }
                    frame "Boolean" {
                      n221 = for {
                        tunnel: [w638] -> w631 mode=indexing
                        tunnel: w629 -> [w635] mode=indexing
                        shift-right: [w639] -> w632
                        shift-left: w633 -> [w640]
                        # "Get Array Elements"
                        n222 = call "get text between brackets.vi"("Python String"=w635) -> ("Text Between Brakets"=w634:string)  [unwired: 10 in]
                        n223 = call <userlib>:"String to 1D Array__ogtk.vi"("delimiter (Tab)"=",", "string"=w634) -> ("Array of Strings"=w636:string[])  [unwired: 9 in]
                        n224 = for {
                          tunnel: [w641] -> w638 mode=indexing
                          tunnel: w636 -> [w642] mode=indexing
                          shift-right: [w644] -> w639
                          shift-left: w640 -> [w645]
                          w643 = FALSE  # Boolean Type
                          n225 = Scan From String(input string=w642, error in=w645, default 1=w643) -> (error out=w644:errorcluster, output 1=w641:bool)  [unwired: 2 in, 2 out]
                        }
                      }
                      n226 = To Variant(anything=w631) -> (Variant=w630:variant)
                    }
                    frame "String" {
                      n227 = for {
                        tunnel: [w655] -> w648 mode=indexing
                        tunnel: w646 -> [w652] mode=indexing
                        shift-right: [w656] -> w649
                        shift-left: w650 -> [w657]
                        # "Get Array Elements"
                        n228 = call "get text between brackets.vi"("Python String"=w652) -> ("Text Between Brakets"=w651:string)  [unwired: 10 in]
                        n229 = call <userlib>:"String to 1D Array__ogtk.vi"("delimiter (Tab)"=",", "string"=w651) -> ("Array of Strings"=w653:string[])  [unwired: 9 in]
                        n230 = for {
                          tunnel: [w659] -> w655 mode=indexing
                          tunnel: w653 -> [w658] mode=indexing
                          shift-right: [w662] -> w656
                          shift-left: w657 -> [w662]
                          n231 = call "Extract First Quoted String.vi"("Strip Quotes (FALSE)"=TRUE, "Quoted String"=w658) -> ("First Quoted String"=w660:string)  [unwired: 7 in, 2 out]
                          n232 = call "Unescape Python String.vi"("Escaped Python String"=w660) -> ("Unescaped String"=w659:string)  [unwired: 10 in]
                        }
                      }
                      n233 = To Variant(anything=w648) -> (Variant=w647:variant)
                    }
                    frame "Path" {
                      n234 = for {
                        tunnel: [w672] -> w665 mode=indexing
                        tunnel: w663 -> [w669] mode=indexing
                        shift-right: [w673] -> w666
                        shift-left: w667 -> [w674]
                        # "Get Array Elements"
                        n235 = call "get text between brackets.vi"("Python String"=w669) -> ("Text Between Brakets"=w668:string)  [unwired: 10 in]
                        n236 = call <userlib>:"String to 1D Array__ogtk.vi"("delimiter (Tab)"=",", "string"=w668) -> ("Array of Strings"=w670:string[])  [unwired: 9 in]
                        n237 = for {
                          tunnel: [w675] -> w672 mode=indexing
                          tunnel: w670 -> [w676] mode=indexing
                          shift-right: [w680] -> w673
                          shift-left: w674 -> [w680]
                          n238 = call "Extract First Quoted String.vi"("Strip Quotes (FALSE)"=TRUE, "Quoted String"=w676) -> ("First Quoted String"=w678:string)  [unwired: 7 in, 2 out]
                          n239 = call "Unescape Python String.vi"("Escaped Python String"=w678) -> ("Unescaped String"=w677:string)  [unwired: 10 in]
                          n240 = String To Path(string=w677) -> (path=w675:path)
                        }
                      }
                      n241 = To Variant(anything=w665) -> (Variant=w664:variant)
                    }
                    frame "Cluster" {
                      # "Get Array Element\nvariant data type"
                      n242 = call <userlib>:"Get Array Element TD__ogtk.vi"("error in (no error)"=w688, "Array"=w687) -> ("error out"=w690:errorcluster, "Type Descriptor"=w689:T2)  [unwired: 8 in]
                      n243 = call <userlib>:"Get Default Data from TD__ogtk.vi"("error in (no error)"=w690, "Type Descriptor"=w689) -> ("error out"=w686:errorcluster, "Default VData"=w685:variant)  [unwired: 8 in]
                      n244 = for {
                        tunnel: w685 -> [w697]
                        tunnel: [w695] -> w683 mode=indexing
                        shift-right: [w696] -> w684
                        shift-left: w686 -> [w692]
                        tunnel: w681 -> [w694] mode=indexing
                        n245 = call "Python List to Array of Elements.vi"("error in (no error)"=w692, "Python List"=w694) -> ("error out"=w691:errorcluster, "Elements"=w693:string[])  [unwired: 8 in]
                        n246 = disable-structure shown="Enabled" {
                          disable-tunnel: w691 -> [w703 w717 _]
                          disable-tunnel: w697 -> [w702 w716 _]
                          disable-tunnel: [w701 w715 _] -> w696
                          disable-tunnel: [w700 w714 _] -> w695
                          disable-tunnel: w693 -> [w699 w713 _]
                          frame Disabled {
                            n247 = call "get text between brackets.vi"("Python String"=w699) -> ("Text Between Brakets"=w698:string)  [unwired: 10 in]
                            n248 = call "Get Array Size from Python String.vi"("Python String"=w698) -> ("Array Size"=w704:i32, "Python String out"=w705:string)  [unwired: 9 in]
                            n249 = for "For each cluster element in the array" {
                              N: w704 -> [_]
                              tunnel: [w706] -> w700 mode=indexing
                              tunnel: w702 -> [w709]
                              shift-right: [w711] -> _
                              shift-left: w705 -> [w712]
                              shift-right: [w707] -> w701
                              shift-left: w703 -> [w708]
                              # "Recursive Call"
                              n250 = call "Split cluster or array pyhton string.vi"(11:w712) -> ("offset past element"=w711:i32, "First Element"=w710:string)  [unwired: 6 in, 3 out]
                              n251 = call "Python String to LabVIEW Data (Variant).vi"("error in (no error)"=w708, "type"=w709, "Python String"=w710) -> ("error out"=w707:errorcluster, "LabVIEW Data"=w706:variant)  [unwired: 7 in]
                            }
                          }
                          frame Enabled {
                            n252 = for "For each cluster element in the array" {
                              tunnel: [w720] -> w714 mode=indexing
                              tunnel: w716 -> [w722]
                              shift-right: [w721] -> w715
                              shift-left: w717 -> [w718]
                              tunnel: w713 -> [w719] mode=indexing
                              # "Recursive Call"
                              n253 = call "Python String to LabVIEW Data (Variant).vi"("error in (no error)"=w718, "type"=w722, "Python String"=w719) -> ("error out"=w721:errorcluster, "LabVIEW Data"=w720:variant)  [unwired: 7 in]
                            }
                          }
                          frame Disabled {
                          }
                        }
                      }
                      n254 = To Variant(anything=w683) -> (Variant=w682:variant)
                    }
                  }
                }
              }
            }
          }
        }
        frame "Cluster" {
          n255 = call "Python List to Array of Elements.vi"("error in (no error)"=w728, "Python List"=w729) -> ("error out"=w727:errorcluster, "Elements"=w724:string[])  [unwired: 8 in]
          n256 = case shown="Default" w725 {
            tunnel: [w735 w743] -> w734
            tunnel: w727 -> [w739 w742]
            tunnel: [w739 w741] -> w726
            tunnel: w724 -> [w738 _]
            tunnel: w723 -> [_ w740]
            frame "<Null>", "Variant" {
              # "We're parsing the string data directly, so create an array of Null variants, so that the For Loop can iterate"
              n257 = Array Size(array=w738) -> (size(s)=w737:i32)
              n258 = Initialize Array(variant ("Variant"), w737) -> (w735:variant[])
            }
            frame Default {
              # "A cluster has a finite (and known) number of elements, so we can recurse on each elements from the variant type"
              # "Expand cluster to its elements"
              n259 = call <userlib>:"Cluster to Array of VData__ogtk.vi"("error in (no error)"=w742, "Cluster"=w740) -> ("error out"=w741:errorcluster, "Array of VData"=w743:variant[])  [unwired: 8 in]
            }
          }
          n260 = for {
            shift-right: [w745] -> w731
            shift-left: w726 -> [w744]
            tunnel: w734 -> [w747] mode=indexing
            tunnel: [w746] -> w732 mode=indexing
            tunnel: w724 -> [w748] mode=indexing
            # "Recursive Call"
            n261 = call "Python String to LabVIEW Data (Variant).vi"("error in (no error)"=w744, "type"=w747, "Python String"=w748) -> ("error out"=w745:errorcluster, "LabVIEW Data"=w746:variant)  [unwired: 7 in]
          }
          n262 = call <userlib>:"Array of VData to VCluster__ogtk.vi"("error in (no error)"=w731, "Array"=w732) -> ("error out"=w730:errorcluster, "VCluster"=w733:variant)  [unwired: 8 in]
        }
        frame Default {
          w752 = 1 items=["No error", "Argument error", "Memory is full", "Out of zone", "End of file", "File already open", "Generic file I/O error", "File not found", "File permission error", "Disk is full", "Duplicate path", "Too many files open", "System feature not enabled", "Resource file not found", "Cannot add resource", "Resource not found", "Image not found", "Image memory error", "Pen does not exist", "Config type invalid", "Config token not found", "Config parse error", "Config memory error", "Bad external code format", "Bad external code offset", "External code not present", "Null window", "Destroy window error", "Null menu", "Print aborted", "Bad print record", "Print driver error", "Windows error during printing", "Memory error during printing", "Print dialog error", "Generic print error", "Invalid device refnum", "Device not found", "Device parameter error", "Device unit error", "Cannot open device", "Device call aborted", "Generic error", "Cancelled by user", "Object ID too low", "Object ID too high", "Object not in heap", "Unknown heap", "Unknown object (invalid DefProc)", "Unknown object (DefProc not in table)", "Message out of range", "Invalid (null) method", "Unknown message", "Manager call not supported", "Bad address", "Network operation in progress", "Network operation timed out", "Connection is busy", "Network attribute not supported", "Network error", "Address in use", "System out of memory", "Connection aborted", "Connection refused", "Not connected", "Already connected", "Connection closed", "Initialization error (interapplication manager)", "Bad occurrence", "Wait on unbound occurrence handler", "Occurrence queue overflow", "Datalog type conflict", "Unused", "Unrecognized type (interapplication manager)", "Memory corrupt", "Failed to make temporary DLL", "Old CIN version", "Drag socket not found", "Failed to load drop-object", "Failed to register OLE object", "Failed to release OLE object", "Format specifier type mismatch", "Unknown format specifier", "Too few format specifiers", "Too many format specifiers", "Scan failed", "Newer CIN version", "Error converting to variant", "Runtime menu error", "Password tampered", "Variant attribute not found", "Incompatible variant data type", "Event data is not available", "Event Store is not present", "Occurrence is not found", "Event Queue is not created", "Event info is not available", "Refnum passed is NULL", "Error retrieving Class GUID", "Error retrieving CoClass GUID", "Error retrieving TypeLib GUID.", "Bad built application magic bytes.", "Specific driver is different from the specific driver associated with the Logical Name.", "There is no session opened to the class driver.", "Max Error", "MAX - Error with config objects", "MAX - Error loading configuration", "MAX - Group not supported"]
          n263 = Format Into String(format string="Unexpected Datatype <%s>" ("Format String"), w749) -> (resulting string=w750:string)  [unwired: 2 in, 1 out]
          n264 = call <userlib>:"Build Error Cluster__ogtk.vi"("String to Prepend to source (\"\")"=w750, "code"=w752) -> ("error out"=w753:errorcluster)
        }
      }
      n265 = call <userlib>:"Set Data Name__ogtk.vi"("error in (no error)"=w12, "Data Name"=w10, "Data"=w11) -> ("error out"=w13:errorcluster, "Renamed Data"=w14:variant)  [unwired: 7 in]
    }
    frame Error {
    }
  }
  "error out" <- w1
  "LabVIEW Data" <- w2
